vi "poly_global_eco_plus.vi"(4 "code (w/out ECO)":i32) -> (1 "code (+ ECO)":i32)   [LabVIEW 2015, in "_error_tools_polys.lvlib"]
uses:
  _error_tools_polys.lvlib
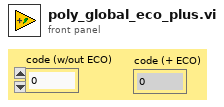
[diagram p1: front panel]
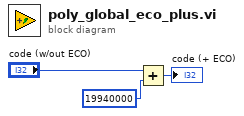
[diagram p0: block diagram]
diagram:
  n1 = Add(x="code (w/out ECO)", y=19940000) -> (x+y=→"code (+ ECO)":i32)
